vi "test RTs Only.vi"(8 "error in":errorcluster, 11 "TestCase in":refnum<class "Create Execution Unit.lvclass">) -> (0 "error out":errorcluster, 3 "TestCase out":refnum<class "Create Execution Unit.lvclass">)   [LabVIEW 2020, in "Create Execution Unit.lvclass"]
uses:
  Create Execution Unit.lvclass
  C:/dev/git/niveristand-custom-device-testing-tools/VeriStandScriptingTestCase/VeriStandScriptingTestCase.lvclass
  Shared/Address.ctl
  niveristand-custom-device-testing-tools/VeriStandScriptingTestCase/VeriStandScriptingTestCase.lvclass/VeriStandScriptingTestCase.ctl
  niveristand-custom-device-testing-tools/VeriStandScriptingTestCase/Read Target.vi
  NationalInstruments.VeriStand.SystemDefinitionAPI
  <vilib>/addons/_JKI Toolkits/VI Tester/TestCase.llb/TestCase.lvclass
  C:/Program Files (x86)/National Instruments/LabVIEW 2020/vi.lib/addons/_JKI Toolkits/VI Tester/TestCase.llb/TestCase.lvclass
  C:/dev/git/niveristand-aim-milStd1553-custom-device/Source/Custom Device Support/Tests/Unit/Create Execution Unit/Create Execution Unit.lvclass
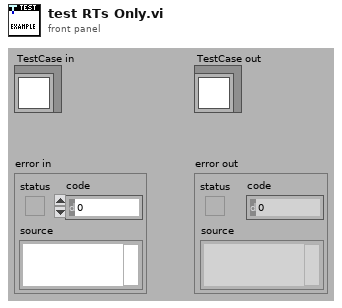
[diagram p1: front panel]
types:
  T1 = typedef "Address.ctl" = u16
  T2 = cluster{"Rx Channel Counts":cluster{"Incoming":i32, "Outgoing":i32, "ReadWrite":i32}, "Rx Message Count":i32, "Tx Acyclic Channel Counts":cluster{"Incoming":i32, "Outgoing":i32, "ReadWrite":i32}, "Triggerable Frames Count":i32, "Tx Channel Counts":cluster{"Incoming":i32, "Outgoing":i32, "ReadWrite":i32}, "Transmitted Message Count":i32, "Expected terminals":T1[], "Expected messages":i32}
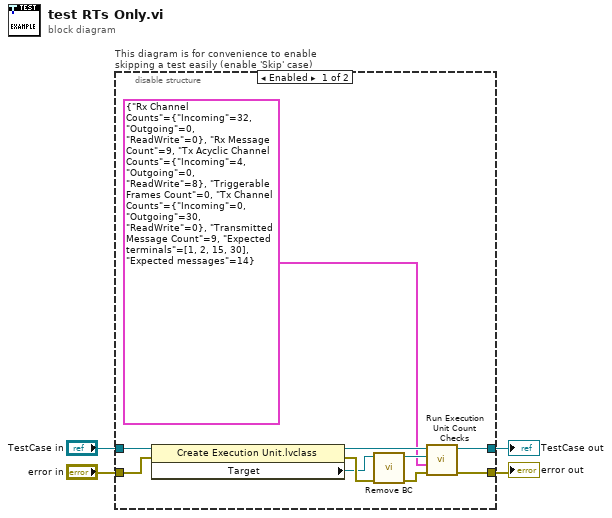
[diagram p0: block diagram]
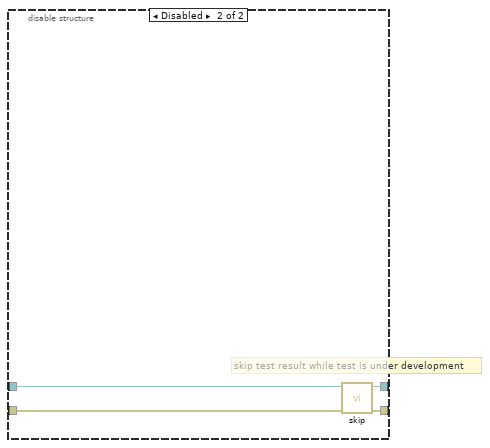
[diagram p2: hidden frame]
diagram:
  n1 = disable-structure "This diagram is for convenience to enable skipping a test easily (enable 'Skip' case)" shown="Enabled" {
    disable-tunnel: "TestCase in" -> [w12 w18]
    disable-tunnel: [w7 w16] -> w1
    disable-tunnel: [w8 w17] -> w3
    disable-tunnel: "error in" -> [w13 w15]
    frame Enabled {
      n2 = property class="Create Execution Unit.lvclass"(reference=w12, error in=w13) -> (reference out=w14:refnum<class "Create Execution Unit.lvclass">, error out=w11:errorcluster, "Target"=w6:refnum<k24>)
      n3 = call "Remove BC.vi"("error in"=w11, "Target in"=w6) -> ("error out"=w10:errorcluster, "Target out"=w9:refnum<k24>)  [unwired: 8 in]
      n4 = call "Run Execution Unit Count Checks.vi"("error in"=w10, "Test Configuration"=T2 {"Rx Channel Counts"={"Incoming"=32, "Outgoing"=0, "ReadWrite"=0}, "Rx Message Count"=9, "Tx Acyclic Channel Counts"={"Incoming"=4, "Outgoing"=0, "ReadWrite"=8}, "Triggerable Frames Count"=0, "Tx Channel Counts"={"Incoming"=0, "Outgoing"=30, "ReadWrite"=0}, "Transmitted Message Count"=9, "Expected terminals"=[1, 2, 15, 30], "Expected messages"=14}, "Target in"=w9, "Create Execution Unit in"=w14) -> ("error out"=w8:errorcluster, "Create Execution Unit out"=w7:refnum<class "Create Execution Unit.lvclass">)  [unwired: 6 in]
    }
    frame Disabled {
      # "skip test result while test is under development"
      n5 = call <vilib>:"skip.vi"("error in (no error)"=w15, "TestCase in"=w18) -> ("error out"=w17:errorcluster, "TestCase out"=w16:refnum<class "Create Execution Unit.lvclass">)  [unwired: 8 in]
    }
  }
  "error out" <- w3
  "TestCase out" <- w1
